vi "Initialize.vi"(8 "error in (no error)":errorcluster, 10 "Top Level Diagram":refnum<vi>, 11 "DMA Loop in":refnum<class "DMA Loop.lvclass">) -> (0 "error out":errorcluster, 3 "DMA Loop out":refnum<class "DMA Loop.lvclass">)   [LabVIEW 2015, in "DMA Loop.lvclass"]
uses:
  DMA Loop.lvclass
  Structures/Structures.lvclass/Structures.ctl
  DMA Loop.lvclass/DMA Loop.ctl
  Structures/Write Structure.vi
  Write Loop Structure.vi
  Structures/Structures.lvclass
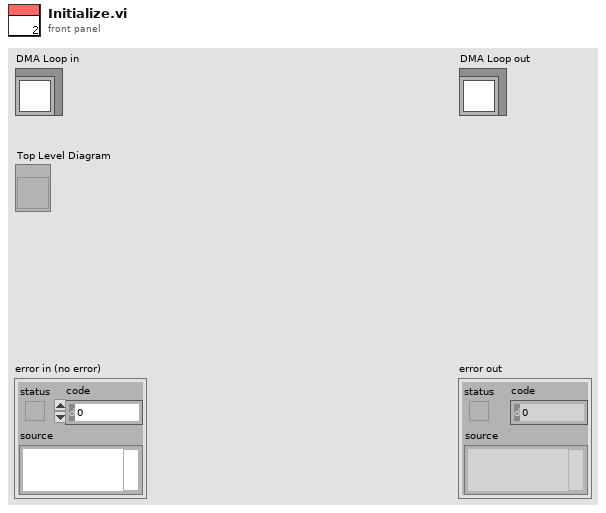
[diagram p1: front panel]
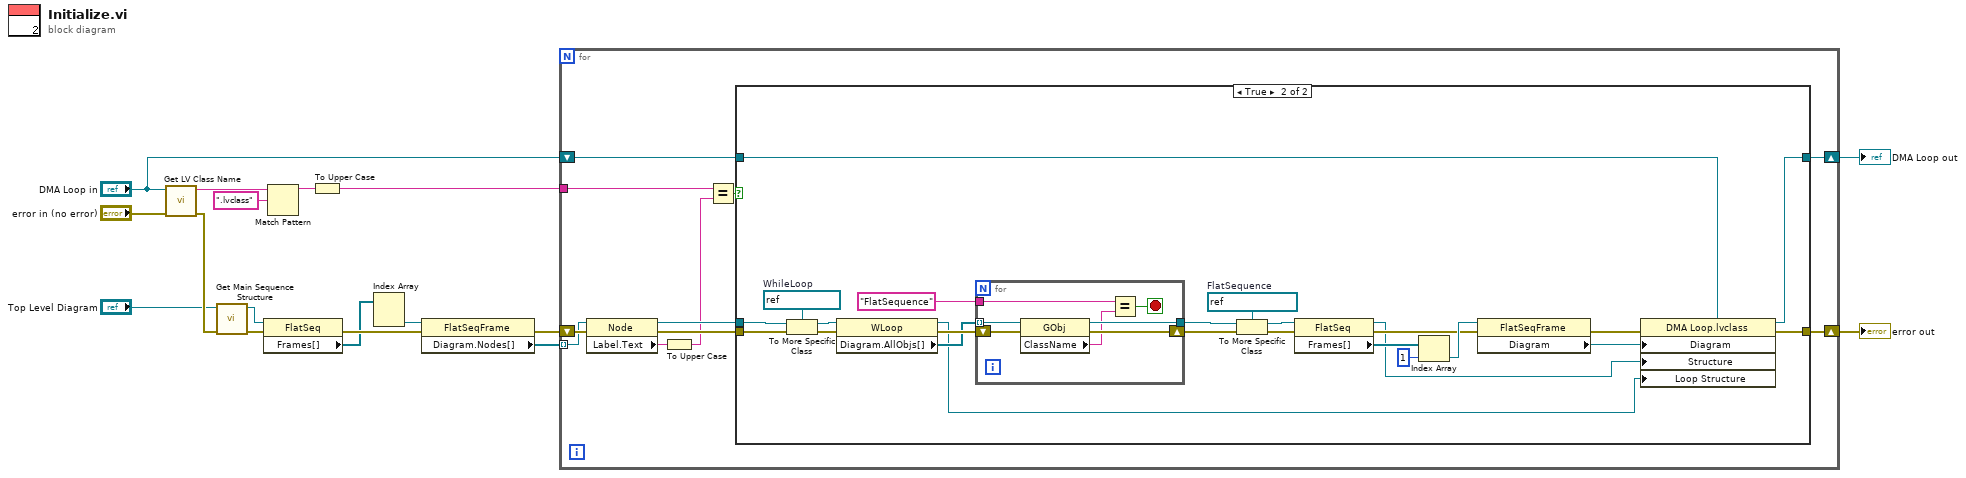
[diagram p0: block diagram]
diagram:
  n1 = call <vilib>:"Get LV Class Name.vi"("error in (no error)"="error in (no error)", "object"="DMA Loop in") -> ("error out"=w8:errorcluster, "class name"=w12:string)  [unwired: 8 in]
  n2 = call "Get Main Sequence Structure.vi"("error in (no error)"=w8, "Top Level Diagram"="Top Level Diagram") -> ("error out"=w7:errorcluster, "Main.SeqStructure"=w6:refnum<vi>)  [unwired: 8 in]
  n3 = property class="FlatSeq"(reference=w6, error in=w7) -> (error out=w14:errorcluster, "Frames[]"=w13:refnum<vi>[])  [unwired: 1 out]
  n4 = Match Pattern(string=w12, regular expression=".lvclass") -> (before substring=w10:string)  [unwired: 1 in, 3 out]
  n5 = To Upper Case(1:w10) -> (0:w9:string)
  n6 = Index Array(array=w13) -> (element #2=w17:refnum<vi>)  [unwired: 2 in, 1 out]
  n7 = property class="FlatSeqFrame"(reference=w17, error in=w14) -> (error out=w16:errorcluster, "Diagram.Nodes[]"=w15:refnum<vi>[])  [unwired: 1 out]
  n8 = for {
    tunnel: w15 -> [w27] mode=indexing
    shift-right: [w23] -> w5
    shift-left: w16 -> [w28]
    tunnel: w9 -> [w21]
    shift-right: [w19] -> w1
    shift-left: "DMA Loop in" -> [w20]
    n9 = property class="Node"(reference=w27, error in=w28) -> (reference out=w25:refnum<vi>, error out=w24:errorcluster, "Label.Text"=w26:string)
    n10 = To Upper Case(1:w26) -> (0:w22:string)
    n11 = Equal?(x=w21, y=w22) -> (x = y?=w18:bool)
    n12 = case shown="True" w18 {
      tunnel: w25 -> [_ w53]
      tunnel: w24 -> [w30 w54]
      tunnel: [w30 w36] -> w23
      tunnel: w20 -> [w29 w33]
      tunnel: [w29 w35] -> w19
      frame False {
      }
      frame True {
        w52 = refnum<vi> refnum  # WhileLoop
        w47 = refnum<vi> refnum  # FlatSequence
        n13 = To More Specific Class(target class=w52, reference=w53, error in=w54) -> (specific class reference=w32:refnum<vi>, error out=w51:errorcluster)
        n14 = property class="WLoop"(reference=w32, error in=w51) -> (reference out=w31:refnum<vi>, error out=w50:errorcluster, "Diagram.AllObjs[]"=w49:refnum<vi>[])
        n15 = for {
          shift-right: [w60] -> w48
          shift-left: w50 -> [w61]
          tunnel: w49 -> [w59] mode=indexing
          tunnel: "FlatSequence" ("name/order") -> [w58]
          tunnel: [w56] -> w45
          stop <- w57 stop-if-true
          n16 = property class="GObj"(reference=w59, error in=w61) -> (reference out=w56:refnum<vi>, error out=w60:errorcluster, "ClassName"=w55:string)
          n17 = Equal?(x=w58, y=w55) -> (x = y?=w57:bool)
        }
        n18 = To More Specific Class(target class=w47, reference=w45, error in=w48) -> (specific class reference=w44:refnum<vi>, error out=w43:errorcluster)
        n19 = property class="FlatSeq"(reference=w44, error in=w43) -> (reference out=w34:refnum<vi>, error out=w40:errorcluster, "Frames[]"=w39:refnum<vi>[])
        n20 = Index Array(array=w39, index=1) -> (element=w41:refnum<vi>)
        n21 = property class="FlatSeqFrame"(reference=w41, error in=w40) -> (error out=w37:errorcluster, "Diagram"=w38:refnum<vi>)  [unwired: 1 out]
        n22 = property class="DMA Loop.lvclass"(reference=w33, error in=w37, "Diagram"=w38, "Structure"=w34, "Loop Structure"=w31) -> (reference out=w35:refnum<class "DMA Loop.lvclass">, error out=w36:errorcluster)
      }
    }
  }
  "error out" <- w5
  "DMA Loop out" <- w1
